vi "pressure_sensor_model.vi"(10 "input_current(V)":dbl) -> (2 "output_pressure(bar)":dbl)   [LabVIEW 2020]
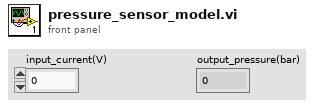
[diagram p1: front panel]
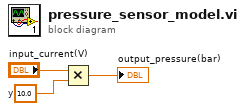
[diagram p0: block diagram]
diagram:
  w2 = 10.0  # y
  n1 = Multiply(x="input_current(V)", y=w2) -> (x*y=→"output_pressure(bar)":dbl)
